vi "Validate TC Parameters.vi"(1 "TC Parameters":T1) -> (0 "Result":T2)   [LabVIEW 2015, in "Config Data.lvlib" / "Config Data.lvclass"]
uses:
  Config Data.lvclass
  Startup Processes/_typedefs/Data Valid Flag.ctl
  Startup Processes/_typedefs/TC Setup Parameters.ctl
  Startup Processes/Startup Processes.lvlib
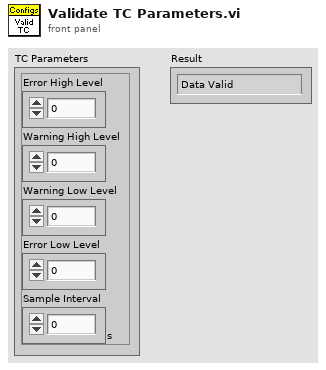
[diagram p1: front panel]
types:
  T1 = typedef "Startup Processes.lvlib/TC Setup Parameters.ctl" = cluster{"Error High Level":dbl, "Warning High Level":dbl, "Warning Low Level":dbl, "Error Low Level":dbl, "Sample Interval":dbl[unit]}
  T2 = typedef "Startup Processes.lvlib/Data Valid Flag.ctl" = enum16{"Data Valid", "Data Not Valid"}
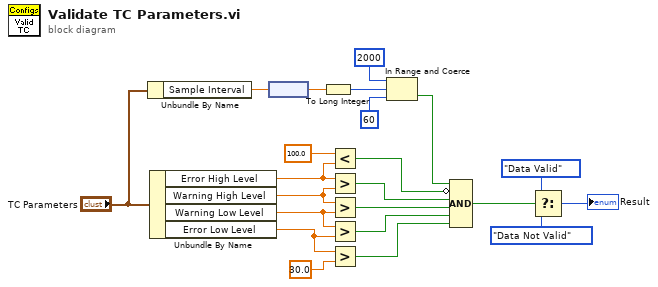
[diagram p0: block diagram]
diagram:
  n1 = Unbundle By Name("TC Parameters") -> ("Sample Interval"=w17:dbl[unit])
  n2 = Unbundle By Name("TC Parameters") -> ("Error High Level"=w7:dbl, "Warning High Level"=w14:dbl, "Warning Low Level"=w13:dbl, "Error Low Level"=w8:dbl)
  n3 = node(w17) -> (w15:dbl)
  n4 = To Long Integer(number=w15) -> (32bit integer=w16:i32)
  n5 = Less?(x=100.0 ("y"), y=w7) -> (x < y?=w5:bool)
  n6 = Greater?(x=w7, y=w14) -> (0:w10:bool)
  n7 = Greater?(x=w14, y=w13) -> (0:w4:bool)
  n8 = Greater?(x=w13, y=w8) -> (0:w3:bool)
  n9 = Greater?(x=w8, y=30.0) -> (0:w2:bool)
  n10 = In Range and Coerce(upper limit=2000, x=w16, lower limit=60 ("upper limit")) -> (In Range?=w1:bool)  [unwired: 1 out]
  n11 = Compound Arithmetic op=AND(w1, invert w5, w10, w4, w3, w2) -> (w12:bool)
  n12 = Select(t=Data_Valid_Flag."Data Valid" ("Enum"), s=w12, f=Data_Valid_Flag."Data Not Valid" ("Enum")) -> (s? t:f=→"Result":T2)
